vi "SUB_Read_specifFile.vi"(3 "name or relative path":string) -> (0 "error out":errorcluster, 1 "text":string)   [LabVIEW 2011]
panel:
  out "path":path
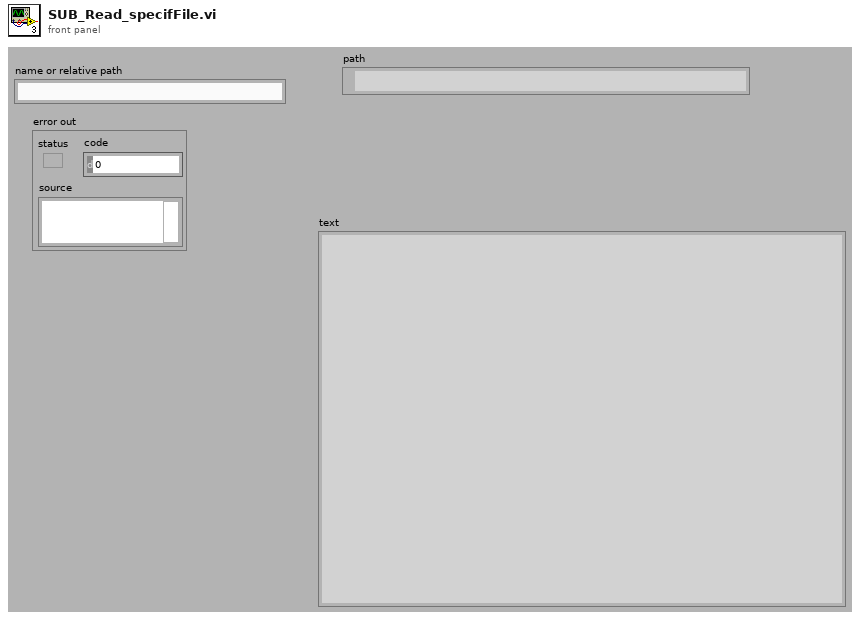
[diagram p1: front panel]
types:
  T1 = enum32{"invalid app kind", "Development System", "Run Time System", "Student Edition", "Embedded LabVIEW", "Evaluation", "Custom"}
  T2 = enum16{"open", "replace", "create", "open or create", "replace or create", "replace or create with confirmation"}
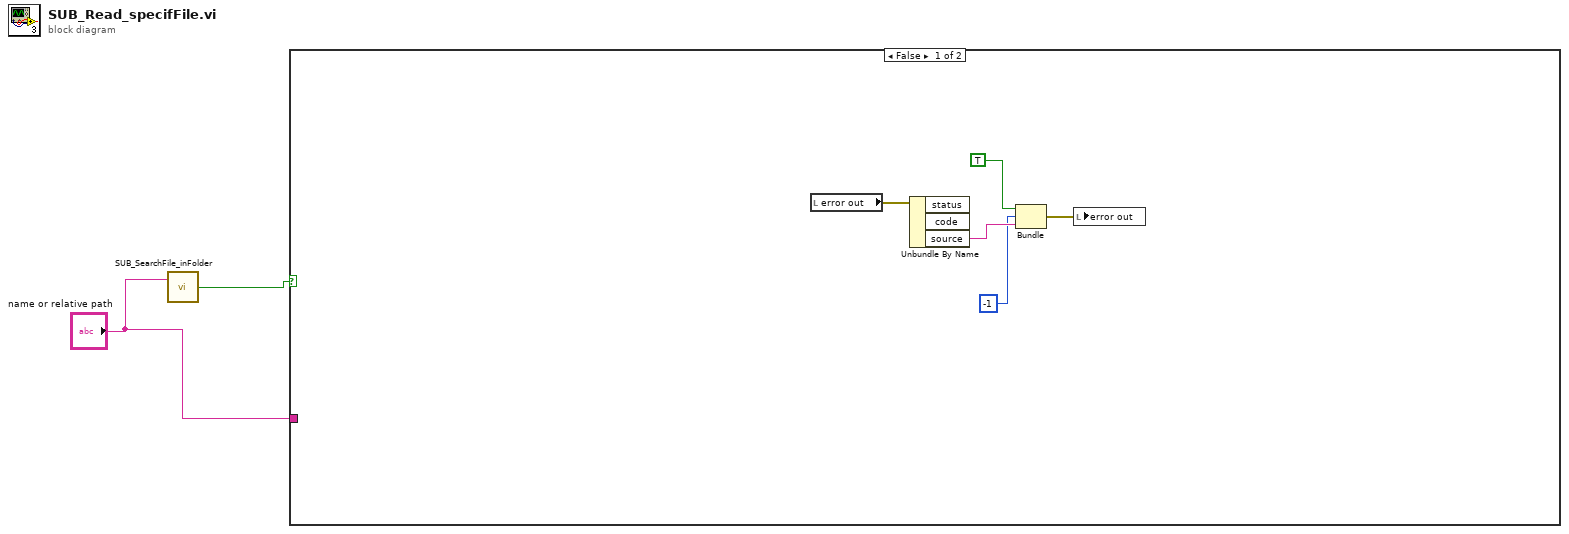
[diagram p0: block diagram]
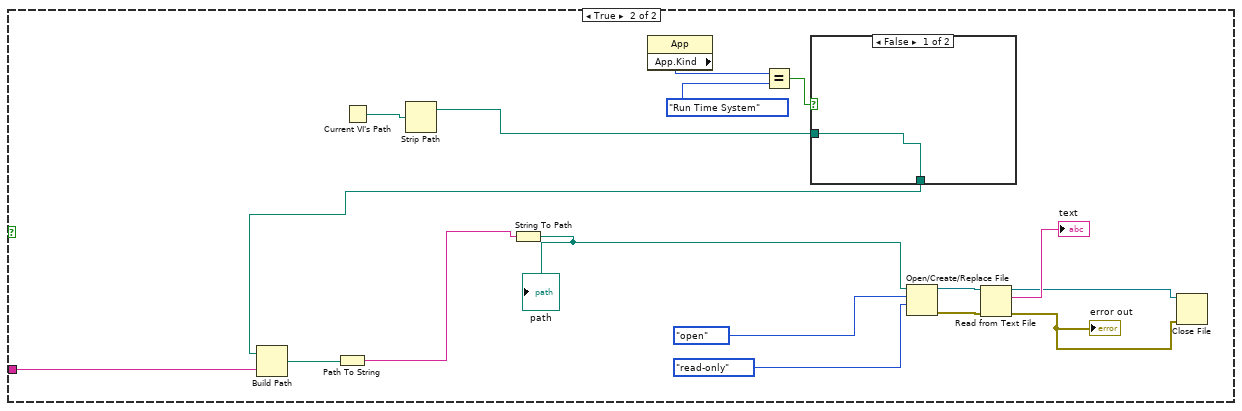
[diagram p2: hidden frame]
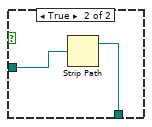
[diagram p3: hidden frame]
diagram:
  n1 = call "SUB_SearchFile_inFolder.vi"("Search Filename in Folder"="name or relative path") -> ("File Existing True/Flase"=w2:bool)  [unwired: 1 in]
  n2 = case shown="False" w2 {
    tunnel: "name or relative path" -> [_ w8]
    frame False {
      n3 = local read "error out"() -> (w7:errorcluster)
      n4 = Unbundle By Name(w7) -> ("source"=w6:string)  [unwired: 2 out]
      n5 = Bundle(TRUE, -1, "source"=w6) -> (w3:cluster{bool, i32, "source":string})  [unwired: 1 in]
      n6 = local write "error out"(w3) -> ()
    }
    frame True {
      n7 = Current VI's Path() -> (path=w19:path)
      n8 = Strip Path(path=w19) -> (stripped path=w15:path)  [unwired: 1 out]
      n9 = property class="App"() -> ("App.Kind"=w18:T1)  [unwired: 2 in, 2 out]
      n10 = Equal?(x=w18, y=T1."Run Time System" ("Application:Kind")) -> (x = y?=w16:bool)
      n11 = case shown="False" w16 {
        tunnel: w15 -> [w25 w27]
        tunnel: [w25 w26] -> w10
        frame False {
        }
        frame True {
          n12 = Strip Path(path=w27) -> (stripped path=w26:path)  [unwired: 1 out]
        }
      }
      n13 = Build Path(base path=w10, name or relative path=w8) -> (appended path=w11:path)
      n14 = Path To String(path=w11) -> (string=w9:string)
      n15 = String To Path(string=w9) -> (path=w14:path)
      "path" <- w14
      n16 = Open/Create/Replace File(file path (use dialog)=w14, operation (0:open)=T2."open", access (0:read/write)=enum16{"read/write", "read-only", "write-only"}."read-only") -> (refnum out=w22:refnum<file>, error out=w21:errorcluster)  [unwired: 3 in, 1 out]
      n17 = Read from Text File(file (use dialog)=w22, error in=w21) -> (refnum out=w13:refnum<file>, text=→"text":string, error out=w12:errorcluster)  [unwired: 2 in, 1 out]
      "error out" <- w12
      n18 = Close File(refnum=w13, error in=w12) -> ()  [unwired: 2 out]
    }
  }
